vi "data-socket.vi"() -> (0 "Price of Liquid Ammonia":dbl)   [LabVIEW 2021]
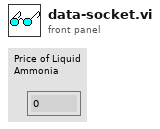
[diagram p1: front panel]
types:
  T1 = enum16{"Read", "Write", "ReadWrite", "BufferedRead", "BufferedReadWrite"}
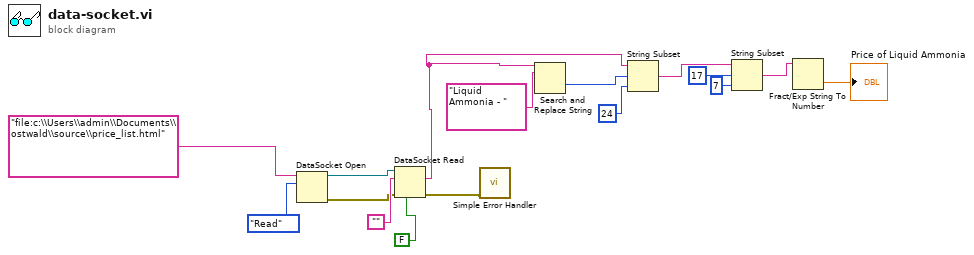
[diagram p0: block diagram]
diagram:
  n1 = DataSocket Open(10:T1."Read" ("mode"), 11:"file:c:\\Users\\admin\\Documents\\ostwald\\source\\price_list.html" ("connection in")) -> (0:w11:errorcluster, 3:w12:refnum<k13>)  [unwired: 2 in]
  n2 = DataSocket Read(6:FALSE ("wait for updated value (T)"), 8:w11, 10:"", 11:w12) -> (0:w13:errorcluster, 2:w7:string)  [unwired: 1 in, 5 out]
  n3 = call <vilib>:"Simple Error Handler.vi"("error in (no error)"=w13) -> ()  [unwired: 4 in, 5 out]
  n4 = Search and Replace String(input string=w7, search string="Liquid Ammonia - ") -> (offset past replacement=w8:i32)  [unwired: 6 in, 3 out]
  n5 = String Subset(string=w7, offset (0)=w8, length (rest)=24 ("length (rest)")) -> (substring=w5:string)
  n6 = String Subset(string=w5, offset (0)=17, length (rest)=7 ("length (rest)")) -> (substring=w1:string)
  n7 = Fract/Exp String To Number(string=w1) -> (number=→"Price of Liquid Ammonia":dbl)  [unwired: 3 in, 1 out]
